vi "OE 1b Factorial (2).vi"() -> ()   [LabVIEW 2021]
panel:
  in  "?":string
  in  "?":string
  in  "Input":dbl
  out "Numeric":i32
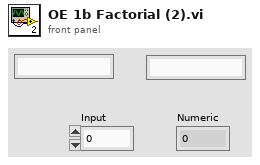
[diagram p1: front panel]
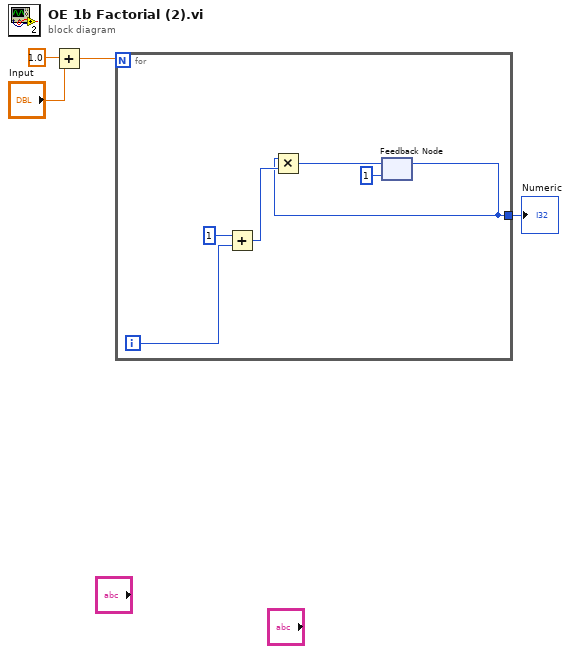
[diagram p0: block diagram]
diagram:
  n1 = Add(x=1.0, y="Input") -> (x+y=w3:dbl)
  n2 = for {
    N: w3 -> [_]
    tunnel: [w6] -> w4
    i -> [w10]
    n3 = Add(x=1, y=w10) -> (x+y=w8:i32)
    n4 = feedback #1(1) -> (w6:i32)
    n5 = Multiply(x=w6, y=w8) -> (x*y=w7:i32)
    n6 = feedback-in #1(w7) -> ()
  }
  "Numeric" <- w4
